vi "Packet_encode_Boolean.vi"(9 "Boolean_Value":bool, 11 "RawData In":u8[](array[numeric])) -> (3 "RawData Out":u8[](array[numeric]))   [LabVIEW 2019, in "PhotonVisionLib.lvlib"]
doc: "Encode (or append) a boolean to the end of an array of bytes. The boolean is stored as an unsigned integer byte, where TRUE = 1, FALSE = 0. \n\nInputs\n - RawData In -- Array of bytes to be appended to..\n - Boolean_Value -- Boolean value.\n\nOutputs\n - RawData Out -- Array of bytes containing the appended value."
uses:
  PhotonVisionLib.lvlib
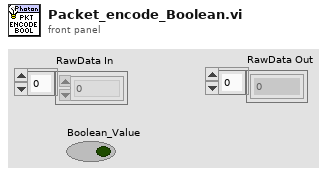
[diagram p1: front panel]
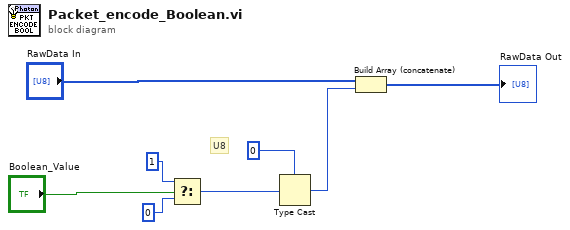
[diagram p0: block diagram]
diagram:
  # "U8"
  n1 = Select(t=u8 1, s="Boolean_Value", f=u8 0) -> (s? t:f=w4:u8)
  n2 = Type Cast(type=u8 0, x=w4) -> (*(type *) &x=w8:u8)
  n3 = Build Array (concatenate)("RawData In", w8) -> (→"RawData Out":u8[])
